vi "end_sCMOS_comms.vi"(0 "sCMOS init":cluster{"init":i16, "sCMOS handle":u32}) -> ()   [LabVIEW 2015]
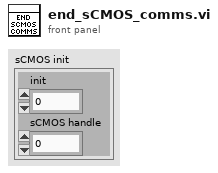
[diagram p1: front panel]
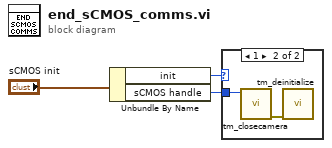
[diagram p0: block diagram]
diagram:
  n1 = Unbundle By Name("sCMOS init") -> ("init"=w2:i16, "sCMOS handle"=w3:u32)
  n2 = case shown="1" w2 {
    tunnel: w3 -> [_ w4]
    frame 0, Default {
    }
    frame 1 {
      n3 = call <userlib>:"tm_closecamera.vi"("Handle in"=w4) -> ("error out"=w5:errorcluster)  [unwired: 10 in]
      n4 = call <userlib>:"tm_deinitialize.vi"("error in (no error)"=w5) -> ()  [unwired: 10 in, 1 out]
    }
  }
